vi "timestamp2sec.vi"(1 "Laptime":timestamp) -> (0 "seconds":dbl)   [LabVIEW 2017]
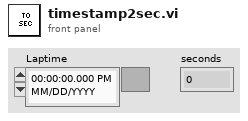
[diagram p1: front panel]
types:
  T1 = typedef "LVDateTimeRec.ctl" = cluster{"fractional second":dbl, "second":i32, "minute":i32, "hour":i32, "day of month":i32, "month":i32, "year":i32, "day of week":i32, "day of year":i32, "DST":i32}
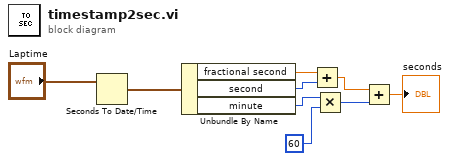
[diagram p0: block diagram]
diagram:
  n1 = Seconds To Date/Time(time stamp (now)="Laptime") -> (date time rec=w2:T1)  [unwired: 1 in]
  n2 = Unbundle By Name(w2) -> ("fractional second"=w3:dbl, "second"=w4:i32, "minute"=w7:i32)
  n3 = Add(x=w3, y=w4) -> (x+y=w5:dbl)
  n4 = Multiply(x=w7, y=60) -> (x*y=w6:i32)
  n5 = Add(x=w5, y=w6) -> (x+y=→"seconds":dbl)
